vi "Load Shared Variable File.vi"(8 "error in":errorcluster, 11 "Device Ref in":T1 format="%.0x") -> (0 "error out":errorcluster, 3 "Device Ref out":T1 format="%.0x")   [LabVIEW 2015, in "Shared Variable Custom Device.lvlib"]
uses:
  Shared Variable Custom Device.lvlib
  <vilib>/NI Veristand/Custom Device API/Custom Device Item Ref.ctl
  <vilib>/Utility/VariantDataType/Type.ctl
  <vilib>/NI Veristand/Custom Device API/Custom Device Channel.ctl
  <vilib>/NI Veristand/Custom Device API/Custom Device Channel Type.ctl
  <userlib>/_OpenG.lib/file/file.llb/Valid Path - Traditional__ogtk.vi
  Shared/Shared Variable GUID Lookup.vi
  Shared/Shared Variable Globals.vi
  <vilib>/Utility/VariantDataType/VariantType.lvlib
  <vilib>/NI Veristand/Custom Device API/Custom Device API.lvlib
panel:
  in  "Cancel Button":bool
  in  "OK Button":bool
  in  "Shared Variable File Path":path
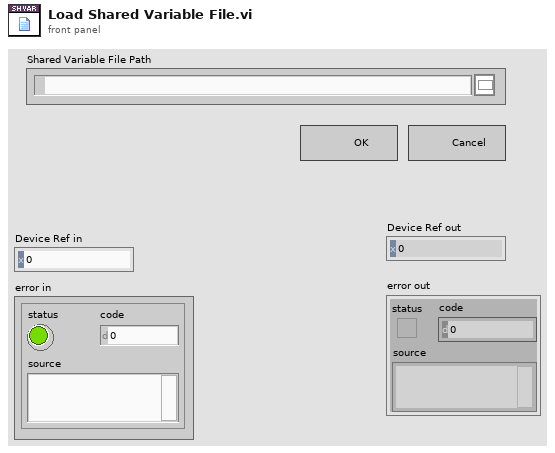
[diagram p1: front panel]
types:
  T1 = typedef "Custom Device API.lvlib/Custom Device Item Ref.ctl" = u64
  T2 = typedef "Custom Device API.lvlib/Custom Device Channel.ctl" = cluster{"Type":T3, "Units":string, "Default Value":dbl, "Faultable":bool, "Scalable":bool}
  T3 = typedef "Custom Device API.lvlib/Custom Device Channel Type.ctl" = enum16{"Input", "Output"}
  T4 = typedef "VariantType.lvlib/Type.ctl" = enum8{"Invalid Type", "Void", "I8", "I16", "I32", "I64", "U8", "U16", "U32", "U64", "Single Float", "Double Float", "Extended Float", "Single Complex", "Double Complex", "Extended Complex", "Enum U8", "Enum U16", "Enum U32", "Enum U64", "Single Float With Unit", "Double Float With Unit", "Extended Float With Unit", "Single Complex with Unit", "Double Complex with Unit", "Extended Complex with Unit", "Boolean", "String", "Path", "Picture", "Tag", "Array", "Cluster", "Variant", "LV Variant", "Waveform", "Timestamp", "Digital Waveform", "Digital Data", "ExpressData", "Refnum", "External Data", "VI", "Poly VI", "LabVIEW Class Instance", "Fixed Point"}
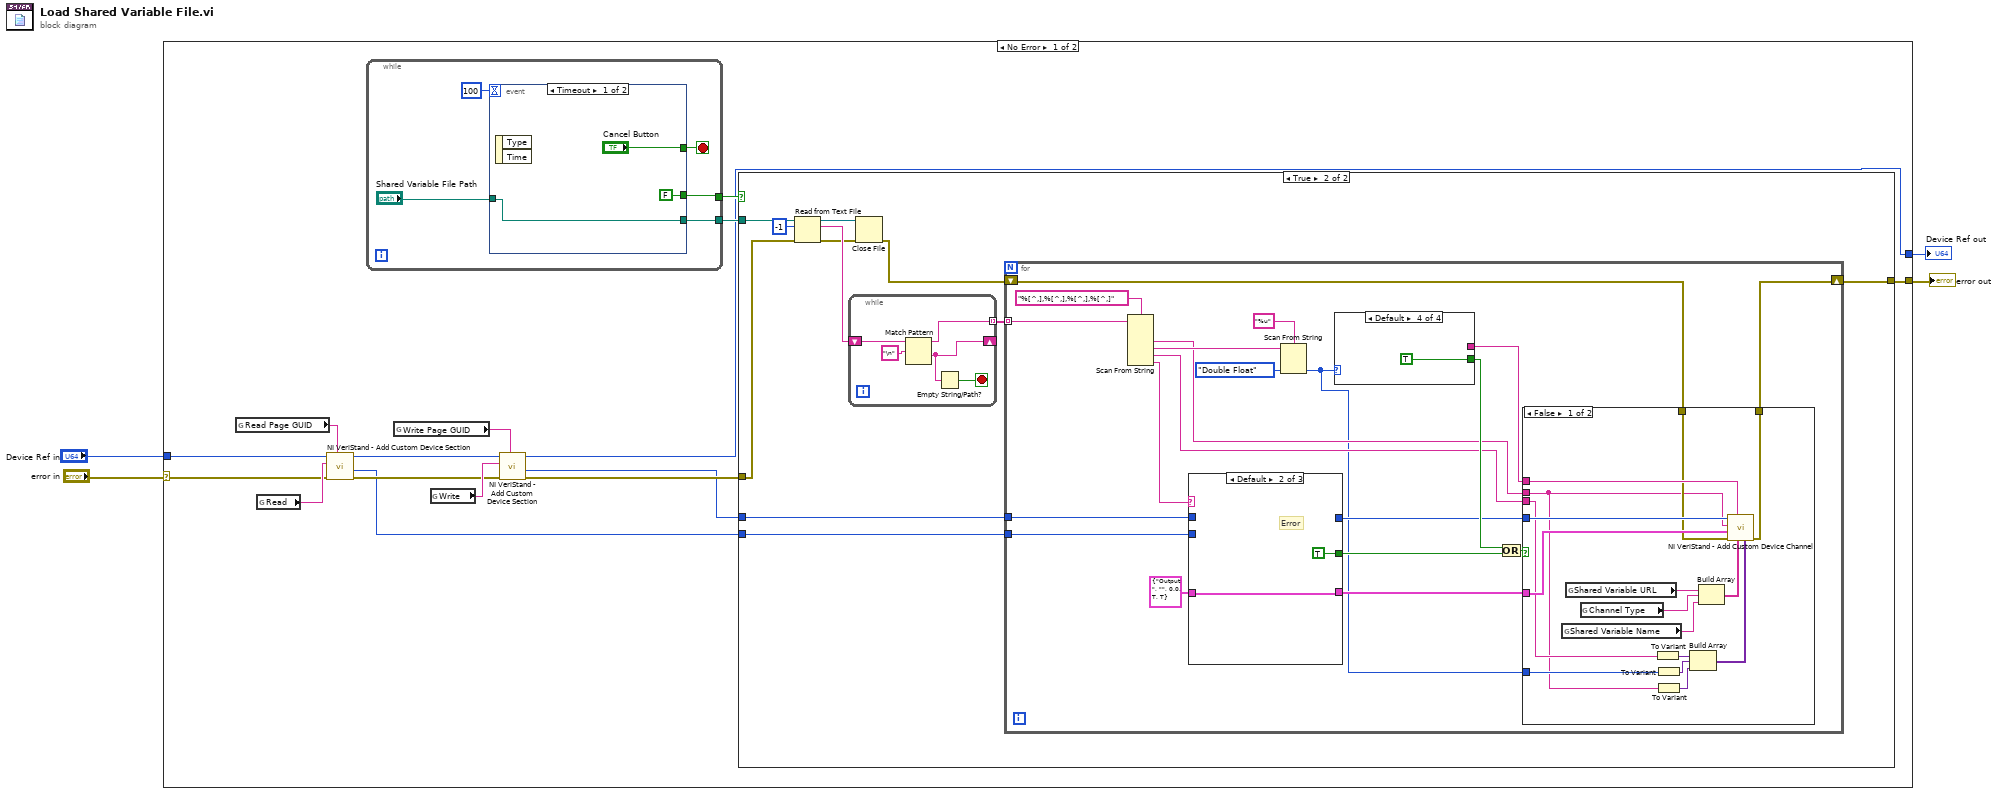
[diagram p0: block diagram]
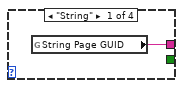
[diagram p3: hidden frame]
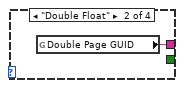
[diagram p4: hidden frame]
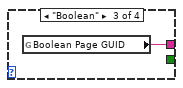
[diagram p5: hidden frame]
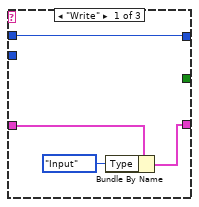
[diagram p7: hidden frame]
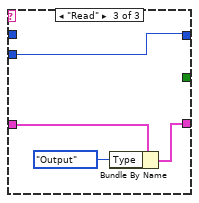
[diagram p8: hidden frame]
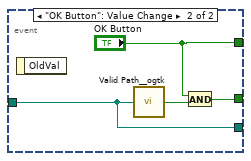
[diagram p9: hidden frame]
diagram:
  n1 = case shown="No Error" "error in" {
    selector: "error in" -> [w6 w101]
    tunnel: "Device Ref in" -> [w11 w100]
    tunnel: [w7 w101] -> w3
    tunnel: [w5 w100] -> w1
    frame No Error {
      n2 = global read "Shared Variable GUID Lookup.vi" "Read Page GUID"() -> (w15:string)
      n3 = global read "Shared Variable Globals.vi" "Read"() -> (w14:string)
      n4 = call <vilib>:"NI VeriStand - Add Custom Device Section.vi"("GUID (Default Section)"=w15, "error in (no error)"=w6, "Section Name"=w14, "Parent Ref in"=w11) -> ("error out"=w13:errorcluster, "Section Ptr"=w9:T1, "Parent Ref out"=w10:T1)  [unwired: 4 in, 1 out]
      n5 = while {
        tunnel: [w89] -> w18
        tunnel: [w88] -> w19
        stop <- w90 stop-if-true
        n6 = event shown="[0] Timeout" {
          selector: _ -> [_ _]
          dyn-events: _ -> [_ _]
          timeout: 100 -> [_ _]
          tunnel: "Shared Variable File Path" -> [w93 w96]
          tunnel: [FALSE w98] -> w88
          tunnel: ["Cancel Button" "OK Button"] -> w90
          tunnel: [w93 w96] -> w89
          event Timeout {
            n7 = event-data() -> ()  [unwired: 1 in, 2 out]
          }
          event "OK Button": Value Change {
            n8 = event-data() -> ()  [unwired: 1 in, 1 out]
            n9 = call-poly <userlib>:"Valid Path__ogtk.vi"("path"=w96) -> ("valid"=w99:bool)
            n10 = And(x="OK Button", y=w99) -> (x .and. y?=w98:bool)
          }
        }
      }
      n11 = global read "Shared Variable GUID Lookup.vi" "Write Page GUID"() -> (w16:string)
      n12 = global read "Shared Variable Globals.vi" "Write"() -> (w17:string)
      n13 = call <vilib>:"NI VeriStand - Add Custom Device Section.vi"("GUID (Default Section)"=w16, "error in (no error)"=w13, "Section Name"=w17, "Parent Ref in"=w10) -> ("error out"=w12:errorcluster, "Section Ptr"=w8:T1, "Parent Ref out"=w5:T1)  [unwired: 4 in, 1 out]
      n14 = case shown="True" w19 {
        tunnel: w18 -> [_ w31]
        tunnel: w12 -> [w20 w29]
        tunnel: w9 -> [_ w23]
        tunnel: w8 -> [_ w24]
        tunnel: [w20 w21] -> w7
        frame False {
        }
        frame True {
          n15 = Read from Text File(file (use dialog)=w31, count=-1, error in=w29) -> (refnum out=w26:refnum<file>, text=w28:string, error out=w27:errorcluster)  [unwired: 1 in, 1 out]
          n16 = while {
            shift-right: [w84] -> _
            shift-left: w28 -> [w87]
            tunnel: [w85] -> w25 mode=indexing
            stop <- w83 stop-if-true
            n17 = Match Pattern(string=w87, regular expression="\n") -> (before substring=w85:string, after substring=w84:string)  [unwired: 1 in, 2 out]
            n18 = Empty String/Path?(string/path=w84) -> (empty?=w83:bool)
          }
          n19 = Close File(refnum=w26, error in=w27) -> (error out=w22:errorcluster)  [unwired: 1 out]
          n20 = for {
            tunnel: w25 -> [w51] mode=indexing
            tunnel: w24 -> [w44]
            tunnel: w23 -> [w45]
            shift-right: [w32] -> w21
            shift-left: w22 -> [w35]
            n21 = Scan From String(format string="%[^,],%[^,],%[^,],%[^,]", input string=w51) -> (output 1=w38:string, output 2=w47:string, output 3=w34:string, output 4=w46:string)  [unwired: 6 in, 3 out]
            n22 = case shown="Default" w46 {
              tunnel: w45 -> [_ _ w82]
              tunnel: w44 -> [w76 _ _]
              tunnel: [_ TRUE _] -> w42
              tunnel: [w76 _ w82] -> w40
              tunnel: T2 {"Type"=enum."Output", "Units"="", "Default Value"=0.0, "Faultable"=TRUE, "Scalable"=TRUE} ("Channel") -> [w75 w77 w81]
              tunnel: [w73 w77 w79] -> w36
              frame "Write" {
                n23 = Bundle By Name(cluster=w75, "Type"=Custom_Device_Channel_Type."Input") -> (w73:T2)
              }
              frame Default {
                # "Error"
              }
              frame "Read" {
                n24 = Bundle By Name(cluster=w81, "Type"=Custom_Device_Channel_Type."Output") -> (w79:T2)
              }
            }
            n25 = Scan From String(format string="%u", input string=w47, default 1=Type."Double Float" ("Type Enum")) -> (output 1=w33:T4)  [unwired: 2 in, 3 out]
            n26 = case shown="Default" w33 {
              tunnel: [_ _ _ TRUE] -> w43
              tunnel: [w52 w53 w54 _] -> w39
              frame "String" {
                n27 = global read "Shared Variable GUID Lookup.vi" "String Page GUID"() -> (w52:string)
              }
              frame "Double Float" {
                n28 = global read "Shared Variable GUID Lookup.vi" "Double Page GUID"() -> (w53:string)
              }
              frame "Boolean" {
                n29 = global read "Shared Variable GUID Lookup.vi" "Boolean Page GUID"() -> (w54:string)
              }
              frame Default {
              }
            }
            n30 = Or(x=w43, y=w42) -> (x .or. y?=w41:bool)
            n31 = case shown="False" w41 {
              tunnel: w40 -> [w71 _]
              tunnel: w39 -> [w70 _]
              tunnel: w38 -> [w57 _]
              tunnel: w36 -> [w69 _]
              tunnel: w35 -> [w68 w72]
              tunnel: w34 -> [w59 _]
              tunnel: w33 -> [w58 _]
              tunnel: [w56 w72] -> w32
              frame False {
                n32 = global read "Shared Variable Globals.vi" "Shared Variable Name"() -> (w65:string)
                n33 = global read "Shared Variable Globals.vi" "Shared Variable URL"() -> (w67:string)
                n34 = global read "Shared Variable Globals.vi" "Channel Type"() -> (w66:string)
                n35 = To Variant(anything=w59) -> (Variant=w63:variant)
                n36 = To Variant(anything=w58) -> (Variant=w62:variant)
                n37 = To Variant(anything=w57) -> (Variant=w60:variant)
                n38 = Build Array(w63, w62, w60) -> (w61:variant[])
                n39 = Build Array(w67, w66, w65) -> (w64:string[])
                n40 = call <vilib>:"NI VeriStand - Add Custom Device Channel.vi"("Property Values"=w61, "Property names"=w64, "GUID (Default Channel)"=w70, "error in (no error)"=w68, "Channel"=w69, "Channel Name"=w57, "Parent Ref in"=w71) -> ("error out"=w56:errorcluster)  [unwired: 1 in, 3 out]
              }
              frame True {
              }
            }
          }
        }
      }
    }
    frame Error {
    }
  }
  "error out" <- w3
  "Device Ref out" <- w1
